vi "Insertion Jig - Find Start.vi"(8 "rect":T1={"left"=316, "top"=15, "right"=389, "bottom"=52}, 11 "picture":picture) -> (0 "First Column":i32, 3 "Edge Set":i32[](array[numeric]))   [LabVIEW 2013]
panel:
  in  "Edge Set Size":dbl=10.0
  out "sub picture":picture
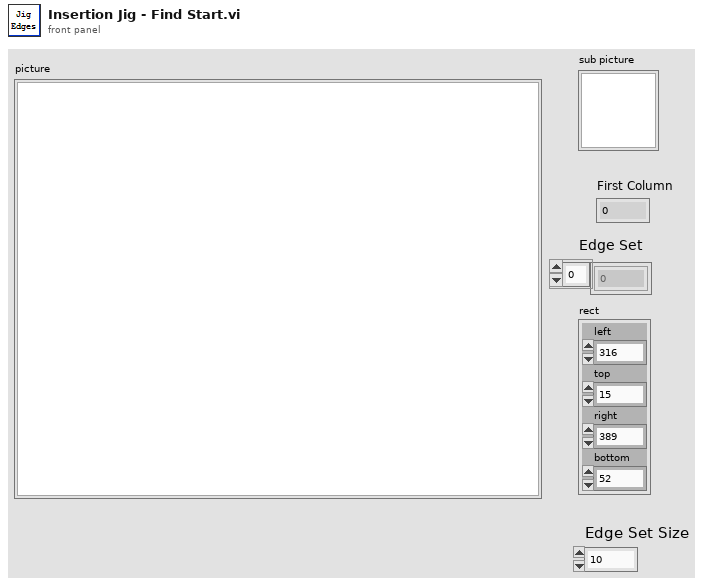
[diagram p1: front panel]
types:
  T1 = cluster{"left":i16, "top":i16, "right":i16, "bottom":i16}
  T2 = typedef "imagedata.ctl" = cluster{"image type":i32, "image depth":i32, "image":u8[], "mask":u8[], "colors":u32[], "Rectangle":cluster{"left":i16, "top":i16, "right":i16, "bottom":i16}}
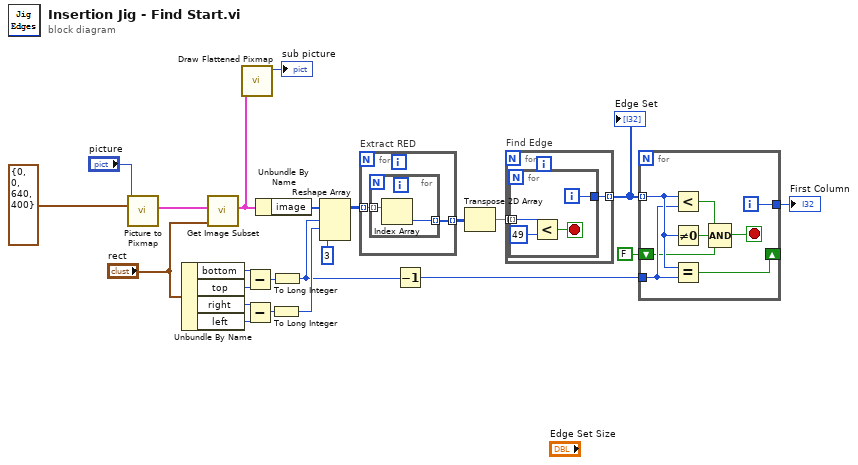
[diagram p0: block diagram]
diagram:
  n1 = call <vilib>:"Picture to Pixmap.vi"("rect"=T1 {"left"=0, "top"=0, "right"=640, "bottom"=400}, "picture"="picture") -> ("image data"=w23:T2)  [unwired: 8 in, 1 out]
  n2 = Unbundle By Name("rect") -> ("bottom"=w16:i16, "top"=w13:i16, "right"=w15:i16, "left"=w14:i16)
  n3 = call <vilib>:"Get Image Subset.vi"("subset rect"="rect", "image data"=w23) -> ("image subset"=w20:T2)  [unwired: 4 in, 1 out]
  n4 = call <vilib>:"Draw Flattened Pixmap.vi"("image data"=w20) -> ("new picture"=→"sub picture":picture)  [unwired: 8 in]
  n5 = Subtract(x=w16, y=w13) -> (x-y=w12:i16)
  n6 = Subtract(x=w15, y=w14) -> (x-y=w11:i16)
  n7 = Unbundle By Name(w20) -> ("image"=w19:u8[])
  n8 = To Long Integer(number=w11) -> (32bit integer=w10:i32)
  n9 = To Long Integer(number=w12) -> (32bit integer=w6:i32)
  n10 = Reshape Array(w19, w6, w10, 3 ("dimension size")) -> (w18:u8[][][])
  n11 = for "Extract RED" {
    tunnel: w18 -> [w25] mode=indexing
    tunnel: [w24] -> w8 mode=indexing
    n12 = for {
      tunnel: w25 -> [w27] mode=indexing
      tunnel: [w26] -> w24 mode=indexing
      n13 = Index Array(array=w27) -> (element=w26:u8)  [unwired: 1 in]
    }
  }
  n14 = Decrement(x=w6) -> (x-1=w5:i32)
  n15 = Transpose 2D Array(2D array=w8) -> (transposed array=w7:u8[][])
  n16 = for "Find Edge" {
    tunnel: w7 -> [w29] mode=indexing
    tunnel: [w28] -> w4 mode=indexing
    n17 = for {
      tunnel: w29 -> [w33] mode=indexing
      tunnel: [w30] -> w28
      i -> [w30]
      stop <- w31 stop-if-true
      n18 = Less?(x=w33, y=u8 49) -> (x < y?=w31:bool)
    }
  }
  "Edge Set" <- w4
  n19 = for {
    tunnel: w5 -> [w38]
    tunnel: w4 -> [w39] mode=indexing
    shift-right: [w41] -> _
    shift-left: FALSE -> [w37]
    tunnel: [w34] -> w2
    i -> [w34]
    stop <- w35 stop-if-true
    n20 = Less?(x=w39, y=w38) -> (x < y?=w36:bool)
    n21 = Not Equal To 0?(x=w39) -> (x != 0?=w40:bool)
    n22 = Equal?(x=w39, y=w38) -> (x = y?=w41:bool)
    n23 = Compound Arithmetic op=AND(w36, w40, w37) -> (w35:bool)
  }
  "First Column" <- w2
